vi "Create.vi"(7 "Direction":T1, 8 "error in (no error)":errorcluster, 9 "Custom Config Data":u8[](array[numeric]), 10 "Name":string, 11 "CIFTag in":refnum<class "CIF_NIChn_Double.lvclass">) -> (0 "error out":errorcluster, 3 "CIFTag out":refnum<class "CIF_NIChn_Double.lvclass">)   [LabVIEW 2021, in "CIF_NIChn_Double.lvclass"]
uses:
  CIF_NIChn_Double.lvclass
  CIF_NIChn_Double.lvclass/CIF_NIChn_Double.ctl
  CIFChannels/CIFChannels.lvclass
  CIFChannels/Typedef/Disconnect Behavior.ctl
  CIFChannels/Typedef/Channel State.ctl
  522c0ff3-de7b-4614-b37e-c276d07c7241.vi
  dcf88837-0f5b-4e9a-81bd-41c3b9e26680.vi
  40444d66-7510-4c55-b376-b17280a77892.vi
  a847dab0-7744-4be7-b05f-57b764edfc6b.vi
  D:/dev/Packages/Channel_Manager/src/CIFChannels/CIFChannels.lvclass
  CIFChannels/Typedef/Direction.ctl
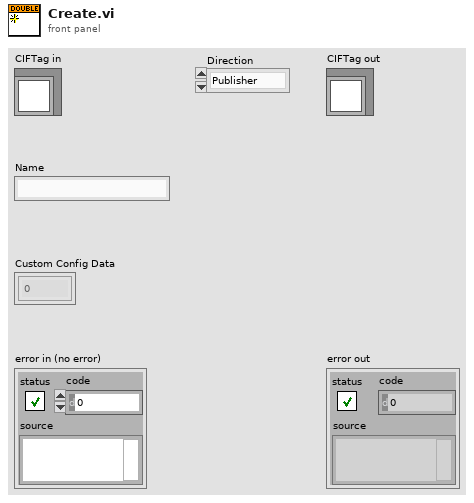
[diagram p1: front panel]
types:
  T1 = typedef "CIFChannels.lvclass/Direction.ctl" = enum16{"Publisher", "Subscriber"}
  T2 = typedef "CIFChannels.lvclass/Disconnect Behavior.ctl" = enum16{"Default value", "Last value", "Error with default"}
  T3 = typedef "CIFChannels.lvclass/Channel State.ctl" = enum16{"Creating", "Disconnected", "Connecting", "Connected", "Destroyed"}
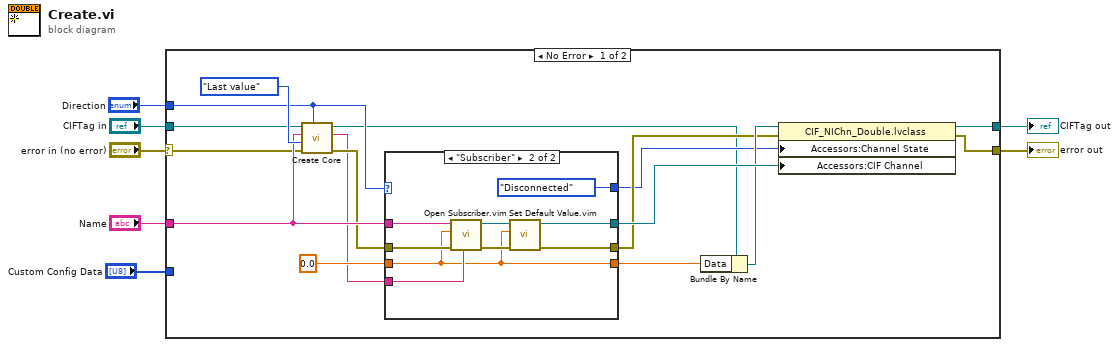
[diagram p0: block diagram]
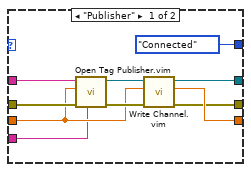
[diagram p2: hidden frame]
diagram:
  n1 = case shown="No Error" "error in (no error)" {
    selector: "error in (no error)" -> [w12 w44]
    tunnel: [w22 w44] -> w1
    tunnel: [w16 w43] -> w5
    tunnel: "CIFTag in" -> [w11 w43]
    tunnel: "Name" -> [w21 _]
    tunnel: "Direction" -> [w15 _]
    tunnel: "Custom Config Data" -> [_ _]
    frame No Error {
      n2 = call "Create Core.vi"("Direction"=w15, "error in (no error)"=w12, "Disconnect Behavior"=Disconnect_Behavior."Last value", "Name"=w21, "CIFChannels in"=w11) -> ("error out"=w10:errorcluster, "Channel Type"=w8:string, "CIFChannels out"=w9:refnum<class "CIF_NIChn_Double.lvclass">)  [unwired: 2 in, 2 out]
      n3 = case shown="\"Subscriber\"" w15 {
        tunnel: w21 -> [w33 w41]
        tunnel: w10 -> [w32 w40]
        tunnel: [w29 w37] -> w20
        tunnel: 0.0 ("Default Value") -> [w28 w34]
        tunnel: [w27 w34] -> w18
        tunnel: [w26 w36] -> w17
        tunnel: w8 -> [w25 w35]
        tunnel: [Channel_State."Connected" ("Channel State") Channel_State."Disconnected" ("Channel State")] -> w14
        frame "Publisher" {
          n4 = call "Open Tag Publisher.vim"("Channel Type Description"=w25, "error in"=w32, "Input Type"=w28, "Channel Name"=w33) -> ("error out"=w30:errorcluster, "CIF Channel"=w31:refnum<k21>)  [unwired: 6 in]
          n5 = call "Write Channel.vim"("error in"=w30, "Data in"=w28, "CIF Channel in"=w31) -> ("error out"=w26:errorcluster, "Data out"=w27:dbl, "CIF Channel out"=w29:refnum<k21>)  [unwired: 5 in, 1 out]
        }
        frame "Subscriber" {
          n6 = call "Open Subscriber.vim"("Channel Type Description"=w35, "error in"=w40, "Input Type"=w34, "Channel Name"=w41) -> ("error out"=w39:errorcluster, "CIF Channel"=w38:refnum<k21>)  [unwired: 6 in]
          n7 = call "Set Default Value.vim"("error in"=w39, "Data in"=w34, "CIF Channel in"=w38) -> ("error out"=w36:errorcluster, "CIF Channel out"=w37:refnum<k21>)  [unwired: 7 in]
        }
      }
      n8 = Bundle By Name(cluster=w9, "Data"=w18) -> (w19:refnum<class "CIF_NIChn_Double.lvclass">)
      n9 = property class="CIF_NIChn_Double.lvclass"(reference=w19, error in=w17, "Accessors:Channel State"=w14, "Accessors:CIF Channel"=w20) -> (reference out=w16:refnum<class "CIF_NIChn_Double.lvclass">, error out=w22:errorcluster)
    }
    frame Error {
    }
  }
  "error out" <- w1
  "CIFTag out" <- w5
